vi "ScanLocationConversionSubVI.vi"(6 "Y Increment":u32, 7 "Y Row Number":u32, 8 "X Increment":u32, 9 "X Row Number":u32, 10 "Data Save Directory:":path=path "C:/Data/test", 11 "File Name:":string="tst8") -> ()   [LabVIEW 2011]
panel:
  out "error out":errorcluster
  out "complete path":path=path "C:/Data/Junk"
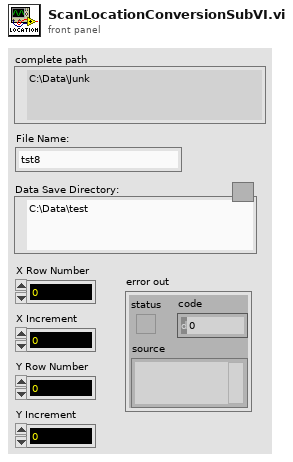
[diagram p1: front panel]
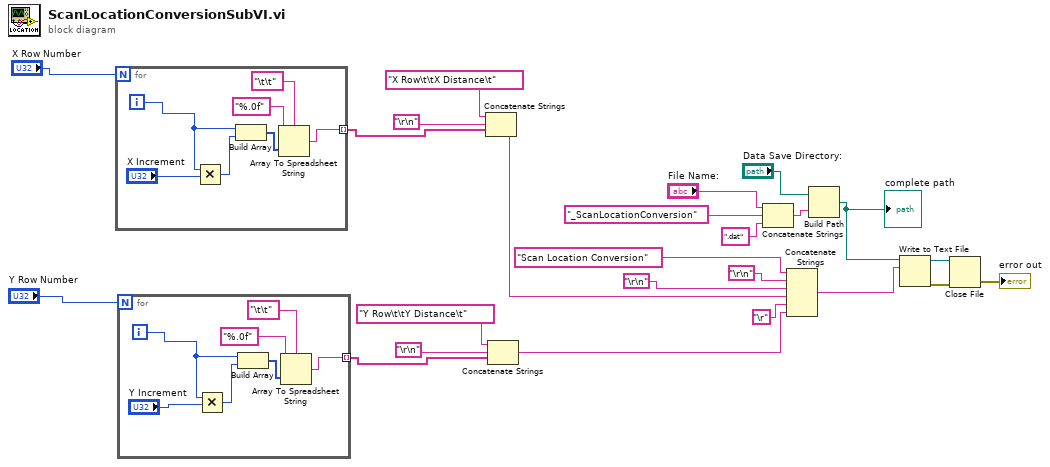
[diagram p0: block diagram]
diagram:
  (unwired) "\r\n"
  n1 = for {
    N: "X Row Number" -> [_]
    tunnel: [w29] -> w11 mode=indexing
    i -> [w27]
    n2 = Multiply(x=w27, y="X Increment") -> (x*y=w26:u32)
    n3 = Build Array(w27, w26) -> (w30:u32[])
    n4 = Array To Spreadsheet String(delimiter (Tab)="\t\t", array=w30, 3:"%.0f") -> (spreadsheet string=w29:string)
  }
  n5 = for {
    N: "Y Row Number" -> [_]
    tunnel: [w36] -> w8 mode=indexing
    i -> [w35]
    n6 = Multiply(x=w35, y="Y Increment") -> (x*y=w34:u32)
    n7 = Build Array(w35, w34) -> (w37:u32[])
    n8 = Array To Spreadsheet String(delimiter (Tab)="\t\t", array=w37, 3:"%.0f") -> (spreadsheet string=w36:string)
  }
  n9 = Concatenate Strings("X Row\t\tX Distance\t", "\r\n", w11) -> (w2:string)
  n10 = Concatenate Strings("Y Row\t\tY Distance\t", "\r\n", w8) -> (w1:string)
  n11 = Concatenate Strings("File Name:", "_ScanLocationConversion", ".dat") -> (w24:string)
  n12 = Concatenate Strings("Scan Location Conversion", "\r\n", "\r\n", w2, "\r", w1) -> (w16:string)
  n13 = Build Path(base path="Data Save Directory:", name or relative path=w24) -> (appended path=w6:path)
  "complete path" <- w6
  n14 = Write to Text File(file (use dialog)=w6, text=w16) -> (refnum out=w18:refnum<file>, error out=w19:errorcluster)  [unwired: 2 in, 1 out]
  n15 = Close File(refnum=w18, error in=w19) -> (error out=→"error out":errorcluster)  [unwired: 1 out]
